vi "Semicolon string to array.vi"(8 "error in":errorcluster, 11 "Semicolon string":string) -> (0 "error out":errorcluster, 3 "String array":string[](array[string]))   [LabVIEW 2012]
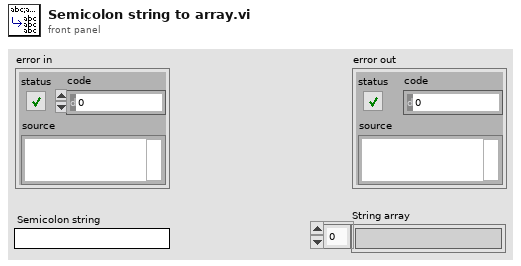
[diagram p1: front panel]
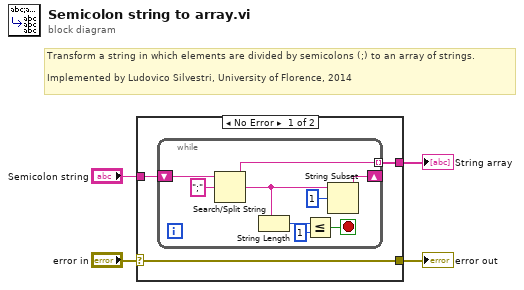
[diagram p0: block diagram]
diagram:
  # "Transform a string in which elements are divided by semicolons (;) to an array of strings. \n\nImplemented by Ludovico Silvestri, University of Florence, 2014"
  n1 = case shown="No Error" "error in" {
    selector: "error in" -> [w5 _]
    tunnel: "Semicolon string" -> [w7 _]
    tunnel: [w6 _] -> w2
    tunnel: [w5 _] -> w1
    frame No Error {
      n2 = while {
        shift-right: [w10] -> _
        shift-left: w7 -> [w16]
        tunnel: [w14] -> w6 mode=indexing
        stop <- w8 stop-if-true
        n3 = Search/Split String(string=w16, search string/char (-)=";") -> (substring before match=w14:string, match + rest of string=w11:string)  [unwired: 1 in, 1 out]
        n4 = String Length(string=w11) -> (length=w13:i32)
        n5 = Less Or Equal?(x=w13, y=1) -> (x <= y?=w8:bool)
        n6 = String Subset(string=w11, offset (0)=1) -> (substring=w10:string)  [unwired: 1 in]
      }
    }
    frame Error {
    }
  }
  "String array" <- w2
  "error out" <- w1
